vi "FilterBias.vi"(6 "dt":dbl, 7 "Graphs":cluster{dbl[], dbl[]}[](array[cluster]), 9 "TargetBias":i32, 10 "Bias":cluster{dbl[], dbl[]}[](array[cluster]), 11 "Show Conductance":bool) -> (3 "Graphs":cluster{dbl[], dbl[]}[](array[cluster]))   [LabVIEW 2024]
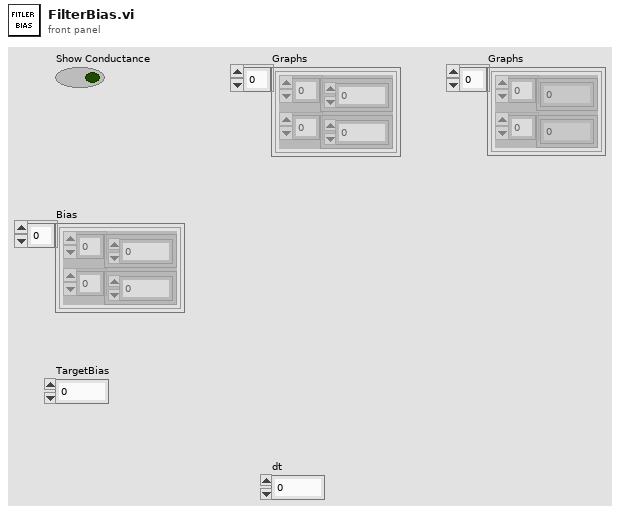
[diagram p1: front panel]
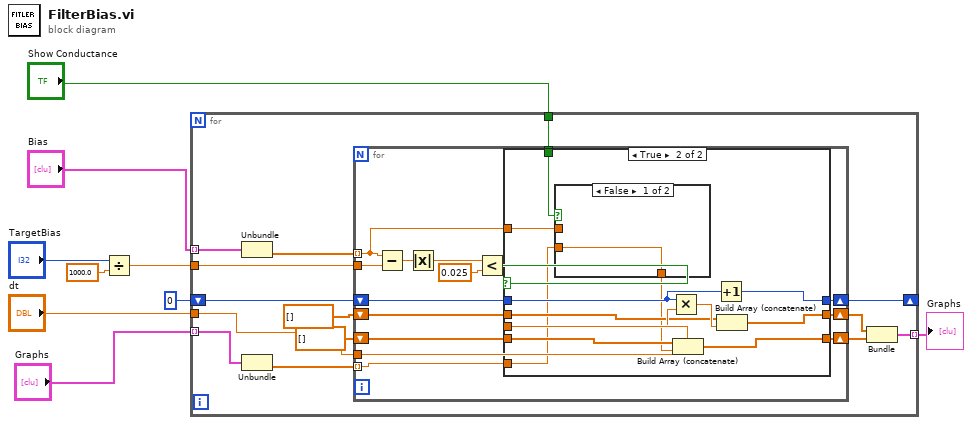
[diagram p0: block diagram]
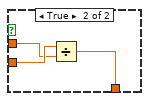
[diagram p3: hidden frame]
diagram:
  n1 = Divide(x="TargetBias", y=1000.0) -> (x/y=w6:dbl)
  n2 = for {
    tunnel: "Bias" -> [w23] mode=indexing
    tunnel: "Graphs" -> [w22] mode=indexing
    tunnel: w6 -> [w19]
    tunnel: [w17] -> w3 mode=indexing
    shift-right: [w14] -> _
    shift-left: 0 -> [w15]
    tunnel: "dt" -> [w13]
    tunnel: "Show Conductance" -> [w10]
    n3 = Unbundle(w23) -> (w21:dbl[])  [unwired: 1 out]
    n4 = Unbundle(w22) -> (w20:dbl[])  [unwired: 1 out]
    n5 = for {
      tunnel: w21 -> [w24] mode=indexing
      tunnel: w20 -> [w33] mode=indexing
      tunnel: w19 -> [w37]
      shift-right: [w32] -> w18
      shift-left: dbl[] [] -> [w31]
      shift-right: [w30] -> w12
      shift-left: dbl[] [] -> [w29]
      tunnel: w13 -> [w26]
      shift-right: [w27] -> w14
      shift-left: w15 -> [w28]
      tunnel: w10 -> [w25]
      n6 = Subtract(x=w24, y=w37) -> (x-y=w38:dbl)
      n7 = Absolute Value(x=w38) -> (abs(x)=w36:dbl)
      n8 = Less?(x=w36, y=0.025) -> (x < y?=w34:bool)
      n9 = case shown="True" w34 {
        tunnel: w33 -> [_ w44]
        tunnel: [w41 w53] -> w32
        tunnel: w31 -> [w41 w52]
        tunnel: [w40 w47] -> w30
        tunnel: w29 -> [w40 w46]
        tunnel: w28 -> [w39 w50]
        tunnel: [w39 w51] -> w27
        tunnel: w26 -> [_ w49]
        tunnel: w25 -> [_ w45]
        tunnel: w24 -> [_ w43]
        frame False {
        }
        frame True {
          n10 = case shown="False" w45 {
            tunnel: w44 -> [w54 w57]
            tunnel: w43 -> [_ w56]
            tunnel: [w54 w55] -> w42
            frame False {
            }
            frame True {
              n11 = Divide(x=w57, y=w56) -> (x/y=w55:dbl)
            }
          }
          n12 = Multiply(x=w50, y=w49) -> (x*y=w48:dbl)
          n13 = Build Array (concatenate)(w52, w42) -> (w53:dbl[])
          n14 = Increment(x=w50) -> (x+1=w51:i32)
          n15 = Build Array (concatenate)(w46, w48) -> (w47:dbl[])
        }
      }
    }
    n16 = Bundle(w12, w18) -> (w17:cluster{dbl[], dbl[]})  [unwired: 1 in]
  }
  "Graphs" <- w3
